vi "trackGlobVarWrite.vi"(0 "stepSize":i32, 1 "start":i32, 2 "nOfSteps":i32, 3 "nOfScans":i32, 4 "invertScan":bool, 5 "heinzingerControl":T1, 9 "waitForKepco(25nsTicks)":u16, 11 "waitAfterReset(25nsTicks)":u16 caption="waitForDmm(25nsTicks)") -> ()   [LabVIEW 2014]
uses:
  Controls/heinzingerSelect.ctl
  <vilib>/rvi/Emulation/niFpgaSctlEmulationGetInTimedLoop.vi
  trackGlobVar.vi
  <vilib>/rvi/Emulation/niFpgaProcessEmulError.vi
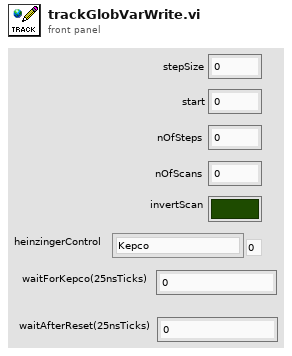
[diagram p1: front panel]
types:
  T1 = typedef "heinzingerSelect.ctl" = enum8{"Kepco", "Heinzinger0", "Heinzinger1", "Heinzinger2"}
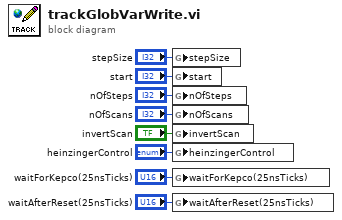
[diagram p0: block diagram]
diagram:
  n1 = global write "trackGlobVar.vi" "stepSize"("stepSize") -> ()
  n2 = global write "trackGlobVar.vi" "start"("start") -> ()
  n3 = global write "trackGlobVar.vi" "nOfSteps"("nOfSteps") -> ()
  n4 = global write "trackGlobVar.vi" "nOfScans"("nOfScans") -> ()
  n5 = global write "trackGlobVar.vi" "invertScan"("invertScan") -> ()
  n6 = global write "trackGlobVar.vi" "heinzingerControl"("heinzingerControl") -> ()
  n7 = global write "trackGlobVar.vi" "waitForKepco(25nsTicks)"("waitForKepco(25nsTicks)") -> ()
  n8 = global write "trackGlobVar.vi" "waitAfterReset(25nsTicks)"("waitAfterReset(25nsTicks)") -> ()
